vi "Set FPGA constants.vi"(8 "error in (no error)":errorcluster, 11 "AODAcq in":refnum<class "AODAcq.lvclass">) -> (0 "error out":errorcluster, 3 "AODAcq out":refnum<class "AODAcq.lvclass">)   [LabVIEW 2014, in "AODAcq.lvclass"]
uses:
  AODAcq.lvclass
  FPGA_Control/AODCalibration.ctl
  AODAcq.lvclass/AODAcq.ctl
  <vilib>/Utility/error.llb/Error Cluster From Error Code.vi
  C:/Program Files (x86)/National Instruments/LabVIEW 2014/Targets/NI/FPGA/StockFPGA_IntfPrivate/ScriptTemplates/StockFPGA_PlugInRead32.vi
  <vilib>/rvi/errors/niLvFpgaAdjustHostInterfaceError.vi
  <vilib>/rvi/interface/nirviReadWriteControl/nirviReadWriteControl.xnode
  FPGA_Control/AODRef.ctl
  FPGA Bitfiles/AodScanner_FPGATarget_AODControl(FPGA)_TyJc9yYmyGA.lvbitx
  NiFpgaLv.dll
  <vilib>/FPGAPlugInAG/PXIe-7965R/niLvFpga_Read32_PXIe-7965R.vi
  <vilib>/rvi/interface/nirviReadWriteControl/niFpgaRWControlAccessTimeoutTemplate.vi
panel:
  in  "AOD.Calibration":T1={"XHP ChirpGain"=1.0, "YHP ChirpGain"=1.0, "XLP ChirpGain"=1.0, "YLP ChirpGain"=1.0}
  in  "AOD.BlankSamples":u16=600
  in  "AOD.ThrowawaySamples":u16=600
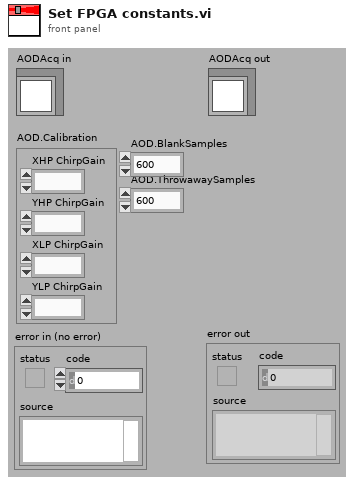
[diagram p1: front panel]
types:
  T1 = typedef "AODCalibration.ctl" = cluster{"XHP ChirpGain":fxp<+/-,16,2>, "YHP ChirpGain":fxp<+/-,16,2>, "XLP ChirpGain":fxp<+/-,16,2>, "YLP ChirpGain":fxp<+/-,16,2>}
  T2 = typedef "AODRef.ctl" = refnum<k20>
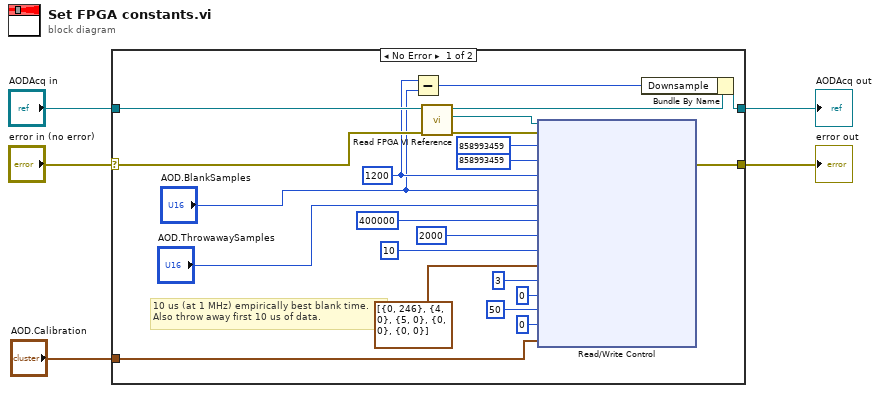
[diagram p0: block diagram]
diagram:
  n1 = case shown="No Error" "error in (no error)" {
    selector: "error in (no error)" -> [w20 w29]
    tunnel: [w19 w29] -> w4
    tunnel: [w7 w28] -> w2
    tunnel: "AODAcq in" -> [w27 w28]
    tunnel: "AOD.Calibration" -> [w6 _]
    frame No Error {
      w11 = u32 1200 ("Downsample")
      # "10 us (at 1 MHz) empirically best blank time.\nAlso throw away first 10 us of data."
      n2 = Subtract(x=w11, y="AOD.BlankSamples") -> (x-y=w8:u32)
      n3 = call-dynamic "Read FPGA VI Reference.vi"("error in (no error)"=w20, "AODAcq in"=w27) -> ("error out"=w25:errorcluster, "FPGA VI Reference"=w26:T2, "AODAcq out"=w9:refnum<class "AODAcq.lvclass">)  [unwired: 7 in]
      n4 = xnode "Read/Write Control"("FPGA VI Reference In"=w26, "error in"=w25, "AOD.HP Center Frequency"=u32 858993459 ("LP Center Frequency"), "AOD.LP Center Frequency"=u32 858993459 ("LP Center Frequency"), "Setup.Downsample"=w11, "AOD.BlankSamples"="AOD.BlankSamples", "AOD.ThrowawaySamples"="AOD.ThrowawaySamples", "Setup.Timeout"=u32 400000 ("Setup.PMT Timeout"), "AOD.UpdatesPerPoint"=u32 2000, "Comm.P high"=u32 10 ("P high"), "Debug.FinishedSetting"=cluster{"Address":u8, "Value":u32}[] [{"Address"=0, "Value"=246}, {"Address"=4, "Value"=0}, {"Address"=5, "Value"=0}, {"Address"=0, "Value"=0}, {"Address"=0, "Value"=0}], "Debug.FinishedSettingSize"=i16 3, "Setup.BitShift"=i16 0, "Comm.UpdateIO time"=u32 50, "Debug.Data"=i16 0 ("Debug Out"), "AOD.Calibration"=w6) -> ("error out"=w19:errorcluster)  [unwired: 1 out]
      n5 = Bundle By Name(cluster=w9, "Downsample"=w8) -> (w7:refnum<class "AODAcq.lvclass">)
    }
    frame Error {
    }
  }
  "error out" <- w4
  "AODAcq out" <- w2
